vi "Build Class Heirarchy.vi"(11 "Classes In":T1(array[cluster])) -> (3 "Classes Out":T1(array[cluster]))   [LabVIEW 2023]
panel:
  out "Array":string[](array[string])
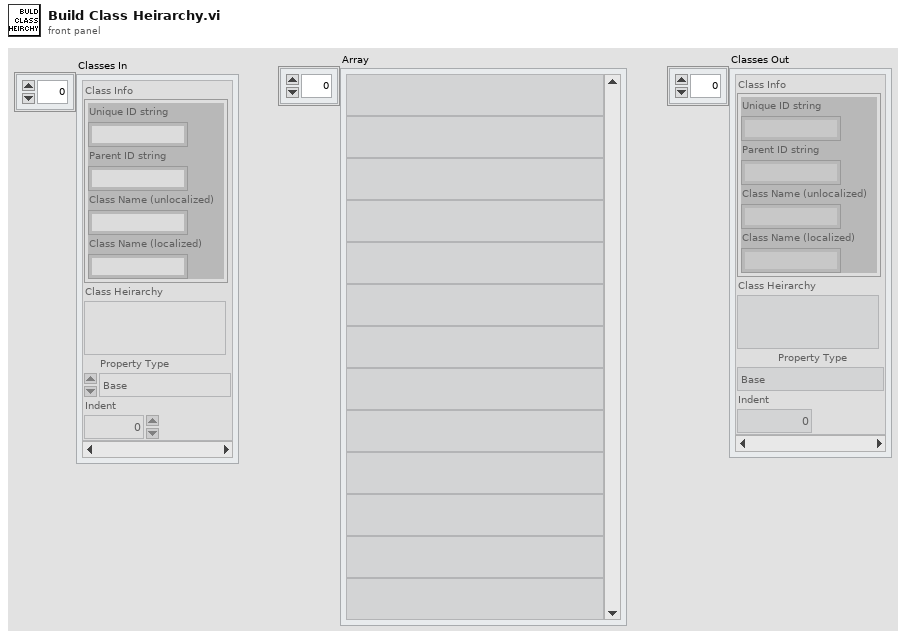
[diagram p1: front panel]
types:
  T1 = cluster{"Class Info":cluster{"Unique ID string":string, "Parent ID string":string, "Class Name (unlocalized)":string, "Class Name (localized)":string}, "Class Heirarchy":string, "Property Type":enum16{"Unknown", "Base", "Scripting", "Private", "Deprecated", "None", "Divider"}, "Indent":u32}[]
  T2 = cluster{"Class Info":cluster{"Unique ID string":string, "Parent ID string":string, "Class Name (unlocalized)":string, "Class Name (localized)":string}, "Class Heirarchy":string, "Property Type":enum16{"Unknown", "Base", "Scripting", "Private", "Deprecated", "None", "Divider"}, "Indent":u32}
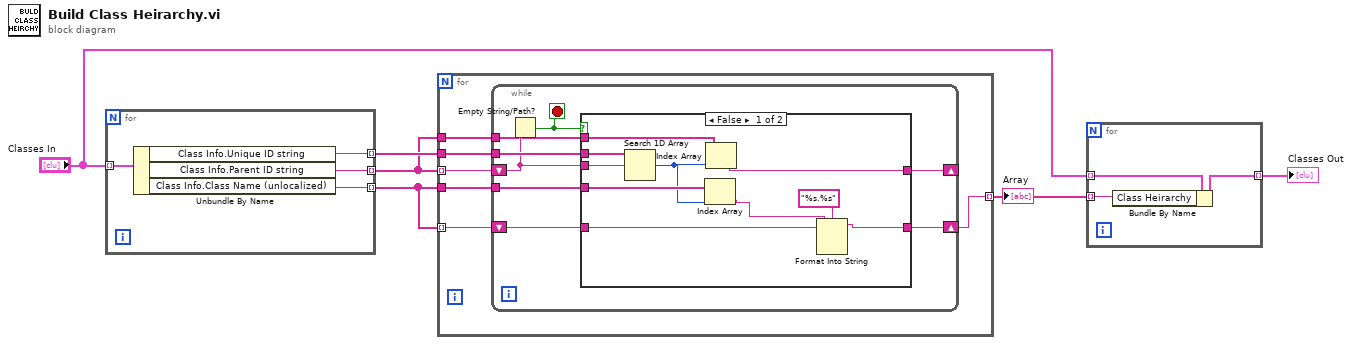
[diagram p0: block diagram]
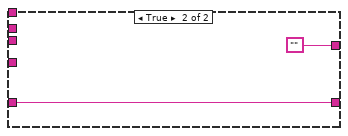
[diagram p2: hidden frame]
diagram:
  n1 = for {
    tunnel: "Classes In" -> [w10] mode=indexing
    tunnel: [w9] -> w6 mode=indexing
    tunnel: [w8] -> w4 mode=indexing
    tunnel: [w7] -> w5 mode=indexing
    n2 = Unbundle By Name(w10) -> ("Class Info.Unique ID string"=w9:string, "Class Info.Parent ID string"=w8:string, "Class Info.Class Name (unlocalized)"=w7:string)
  }
  n3 = for {
    tunnel: w4 -> [w12] mode=indexing
    tunnel: w6 -> [w16]
    tunnel: w5 -> [w15]
    tunnel: w5 -> [w14] mode=indexing
    tunnel: [w13] -> w2 mode=indexing
    tunnel: w4 -> [w11]
    n4 = while {
      tunnel: w16 -> [w24]
      tunnel: w15 -> [w23]
      shift-right: [w21] -> w13
      shift-left: w14 -> [w22]
      shift-right: [w18] -> _
      shift-left: w12 -> [w20]
      tunnel: w11 -> [w17]
      stop <- w19 stop-if-true
      n5 = Empty String/Path?(string/path=w20) -> (empty?=w19:bool)
      n6 = case shown="False" w19 {
        tunnel: w24 -> [w25 _]
        tunnel: w20 -> [w34 _]
        tunnel: w23 -> [w33 _]
        tunnel: w22 -> [w32 w36]
        tunnel: [w29 w36] -> w21
        tunnel: [w27 ""] -> w18
        tunnel: w17 -> [w26 _]
        frame False {
          n7 = Search 1D Array(1D array=w25, element=w34) -> (index of element=w28:i32)  [unwired: 1 in]
          n8 = Index Array(array=w33, index=w28) -> (element=w31:string)
          n9 = Index Array(array=w26, index=w28) -> (element=w27:string)
          n10 = Format Into String(format string="%s.%s", w31, w32) -> (resulting string=w29:string)  [unwired: 2 in, 1 out]
        }
        frame True {
        }
      }
    }
  }
  "Array" <- w2
  n11 = for {
    tunnel: "Classes In" -> [w39] mode=indexing
    tunnel: w2 -> [w38] mode=indexing
    tunnel: [w37] -> w1 mode=indexing
    n12 = Bundle By Name(cluster=w39, "Class Heirarchy"=w38) -> (w37:T2)
  }
  "Classes Out" <- w1
